vi "NovRAM Read.vi"(8 "error in (no error)":errorcluster, 10 "NOVRAM ADDRESS":u8=1 min=1 max=64 step=1, 11 "VISA resource name":refnum<visa-resource-name>) -> (0 "error out":errorcluster, 2 "WORD READ":u16 step=1 format="%.0x", 3 "VISA resource name out":refnum<visa-resource-name>)   [LabVIEW 2023, in "Digikrom DK24x.lvlib"]
doc: "Reads a word (0 to 65535) to a Novram address (1 to 64) indicated by address byte."
uses:
  Digikrom DK24x.lvlib
  Private/Command.ctl
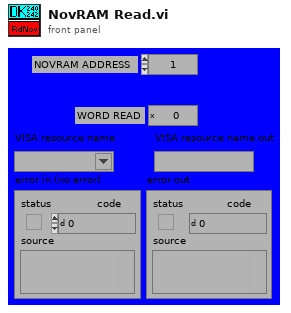
[diagram p1: front panel]
types:
  T1 = typedef "Digikrom DK24x.lvlib/Command.ctl" = u8
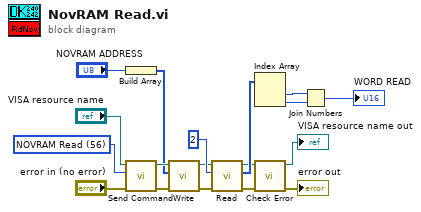
[diagram p0: block diagram]
diagram:
  w1 = T1 56 items=["Cancel"=24, "Clear"=25, "CSR"=28, "Echo"=27, "Filter"=15, "Gcal"=18, "Goto"=16, "Grtid?"=19, "Grtsel"=26, "NOVRAM Read"=56, "NOVRAM Write"=59, "Reset"=255, "Scan"=12, "Scan Up"=9, "Scan Down"=3, "Serial?"=33, "Slew Up"=8, "Slew Down"=2, "Slit Reset"=43, "Slit?"=30, "Sltadj"=14, "Speed"=13, "Sspeed?"=21, "Step Down"=1, "Step Up"=7, "S1adj"=31, "S2adj"=32, "S3adj"=34, "S1cal"=22, "S2cal"=23, "S3cal"=35, "Test"=17, "Type"=57, "Wave?"=29, "Zero"=52] ("Command")
  n1 = Build Array("NOVRAM ADDRESS") -> (w2:u8[])
  n2 = call "Send Command.vi"("error in (no error)"="error in (no error)", "Command"=w1, "VISA resource name"="VISA resource name") -> ("error out"=w6:errorcluster, "VISA resource name out"=w7:refnum<visa-resource-name>)  [unwired: 7 out]
  n3 = call "Write.vi"("error in (no error)"=w6, "Byte Array"=w2, "VISA resource name"=w7) -> ("error out"=w13:errorcluster, "VISA resource name out"=w12:refnum<visa-resource-name>)  [unwired: 7 out]
  n4 = call "Read.vi"("error in (no error)"=w13, "response size"=u8 2, "VISA resource name"=w12) -> ("error out"=w10:errorcluster, "response array"=w17:u8[], "VISA resource name out"=w11:refnum<visa-resource-name>)  [unwired: 6 out]
  n5 = Index Array(array=w17) -> (element #1=w16:u8, element #2=w3:u8)  [unwired: 2 in]
  n6 = call "Check Error.vi"("error in"=w10, "VISA resource name in"=w11) -> ("error out"=→"error out":errorcluster, "VISA resource name out"=→"VISA resource name out":refnum<visa-resource-name>)  [unwired: 1 in, 7 out]
  n7 = Join Numbers(hi=w16, lo=w3) -> ((hi.lo)=→"WORD READ":u16)
